vi "Flicker.vi"() -> ()   [LabVIEW 2014]
uses:
  C:/Users/ThomasNelson/Projects/examples/libraries/bin/visual .net/KClmtrWrapper.dll
  libraries/bin/visual .net/KClmtrWrapper.dll
panel:
  out "Cluster":T1
  in  "Port Number":i32=3
  in  "Stop":bool
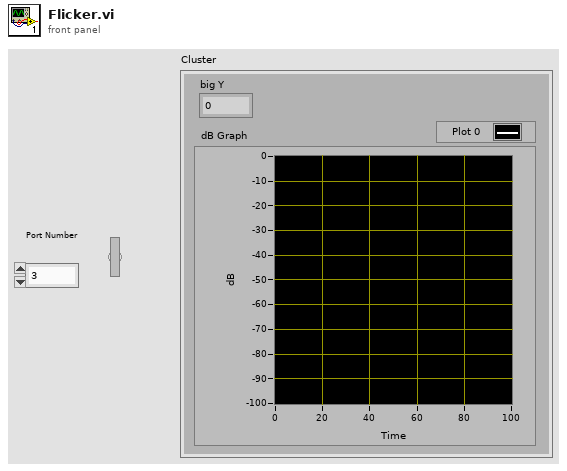
[diagram p1: front panel]
types:
  T1 = cluster{"dB Graph":cluster{"X":dbl, "Y":dbl}[], "big Y":dbl}
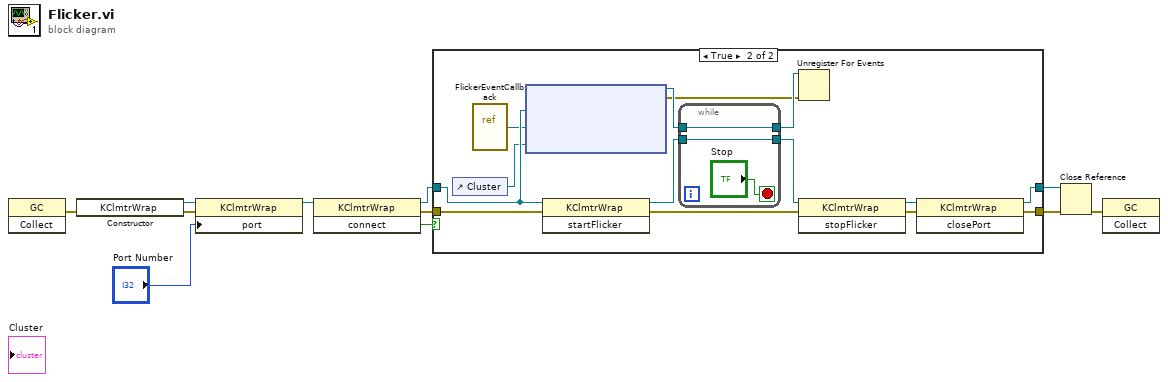
[diagram p0: block diagram]
diagram:
  n1 = invoke class="GC" method="Collect"() -> (error out=w1:errorcluster)  [unwired: 3 in, 2 out]
  n2 = constructor class="KClmtrWrap"(error in=w1) -> (reference out=w11:refnum<k24>, error out=w10:errorcluster)  [unwired: 2 in, 1 out]
  n3 = property class="KClmtrWrap"(reference=w11, error in=w10, "port"="Port Number") -> (reference out=w8:refnum<k24>)  [unwired: 1 out]
  n4 = invoke class="KClmtrWrap" method="connect"(reference=w8) -> (reference out=w5:refnum<k24>, error out=w4:errorcluster, "connect"=w3:bool)  [unwired: 2 in]
  n5 = case shown="True" w3 {
    tunnel: w5 -> [w13 w16]
    tunnel: w4 -> [w12 w19]
    tunnel: [w13 w27] -> w7
    tunnel: [w12 w26] -> w6
    frame False {
    }
    frame True {
      n6 = control-ref of="Cluster"() -> (w15:refnum<vi>)
      n7 = vi-ref "FlickerEventCallback.vi"() -> ("vi reference"=w14:refnum<vi>)
      n8 = node(w16, w14, w15) -> (w22:refnum<k27>, w21:errorcluster)  [unwired: 2 in]
      n9 = invoke class="KClmtrWrap" method="startFlicker"(reference=w16, error in=w19) -> (reference out=w20:refnum<k24>, error out=w25:errorcluster)  [unwired: 1 in, 1 out]
      n10 = while {
        tunnel: w20 -> [w28]
        tunnel: [w29] -> w23
        tunnel: w22 -> [w29]
        tunnel: [w28] -> w17
        stop <- "Stop" stop-if-true
      }
      n11 = Unregister For Events(event registration refnum=w23, error in=w21) -> ()  [unwired: 1 out]
      n12 = invoke class="KClmtrWrap" method="stopFlicker"(reference=w17, error in=w25) -> (reference out=w24:refnum<k24>, error out=w18:errorcluster)  [unwired: 1 in, 1 out]
      n13 = invoke class="KClmtrWrap" method="closePort"(reference=w24, error in=w18) -> (reference out=w27:refnum<k24>, error out=w26:errorcluster)  [unwired: 1 in, 1 out]
    }
  }
  n14 = Close Reference(reference=w7, error in (no error)=w6) -> (error out=w2:errorcluster)
  n15 = invoke class="GC" method="Collect"(error in=w2) -> ()  [unwired: 2 in, 3 out]
